vi "Termometr.vi"() -> ()   [LabVIEW 2023]
uses:
  <vilib>/numeric/Random Number (Range) I64.vi
  <vilib>/numeric/sub_Random U32.vi
panel:
  in  "stop":bool
  in  "Skala temperatury":bool
  out "Temperatura [F]":dbl(slide) scale=0.0..100.0
  out "Temperatura [F]":dbl(slide) scale=0.0..100.0
  # "Deg C"
  # "Deg F"
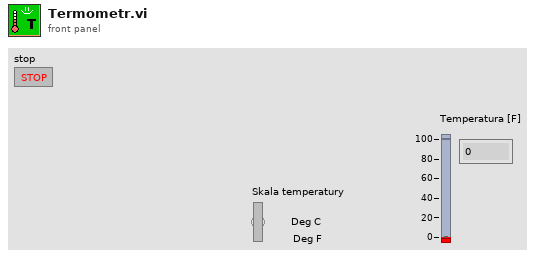
[diagram p1: front panel]
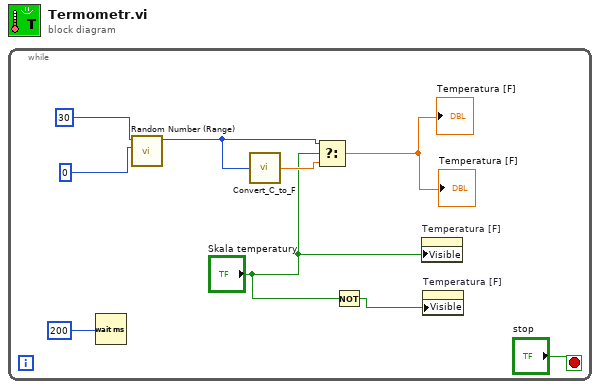
[diagram p0: block diagram]
diagram:
  n1 = while {
    stop <- "stop" stop-if-true
    n2 = Wait (ms)(milliseconds to wait=200) -> ()  [unwired: 1 out]
    n3 = call-poly <vilib>:"Random Number (Range).vi"("lower bound (-100)"=0, "upper bound (100)"=30) -> ("number"=w1:i64)  [unwired: 9 in]
    n4 = call "Convert_C_to_F.vi"("deg C"=w1) -> ("deg F"=w5:dbl)
    n5 = Select(t=w1, s="Skala temperatury", f=w5) -> (s? t:f=→"Temperatura [F]" →"Temperatura [F]":dbl)
    n6 = Not(x="Skala temperatury") -> (.not. x?=w8:bool)
    n7 = property on="Temperatura [F]" class="Slide (strict)"("Visible"="Skala temperatury") -> ()  [unwired: 2 in, 2 out]
    n8 = property on="Temperatura [F]" class="Slide (strict)"("Visible"=w8) -> ()  [unwired: 2 in, 2 out]
  }
